vi "test_Expected Response Trigger - S1.vi"(8 "error in (no error)":errorcluster, 11 "TestCase in":refnum<class "Expected Response Trigger test.lvclass">) -> (0 "error out":errorcluster, 3 "TestCase out":refnum<class "Expected Response Trigger test.lvclass">)   [LabVIEW 2017, in "Expected Response Trigger test.lvclass"]
uses:
  Expected Response Trigger test.lvclass
  Libraries/SSH/Expected Response String Config.ctl
  Libraries/SSH/Search Start Point.ctl
  <vilib>/addons/_JKI Toolkits/VI Tester/TestCase.llb/TestCase.lvclass
  Libraries/SSH/SSH.lvlib
  C:/Program Files (x86)/National Instruments/LabVIEW 2017/vi.lib/addons/_JKI Toolkits/VI Tester/TestCase.llb/TestCase.lvclass
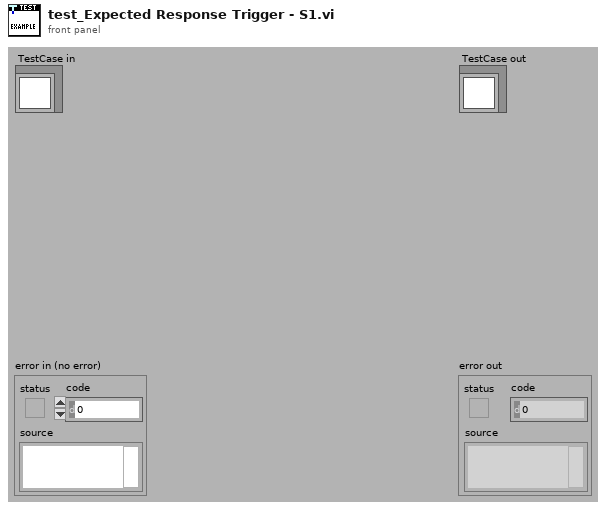
[diagram p1: front panel]
types:
  T1 = typedef "SSH.lvlib/Expected Response String Config.ctl" = cluster{"Expected Response":string, "Search Start Point":T2, "Instance Count":i32}
  T2 = typedef "SSH.lvlib/Search Start Point.ctl" = enum16{"From Start", "From End"}
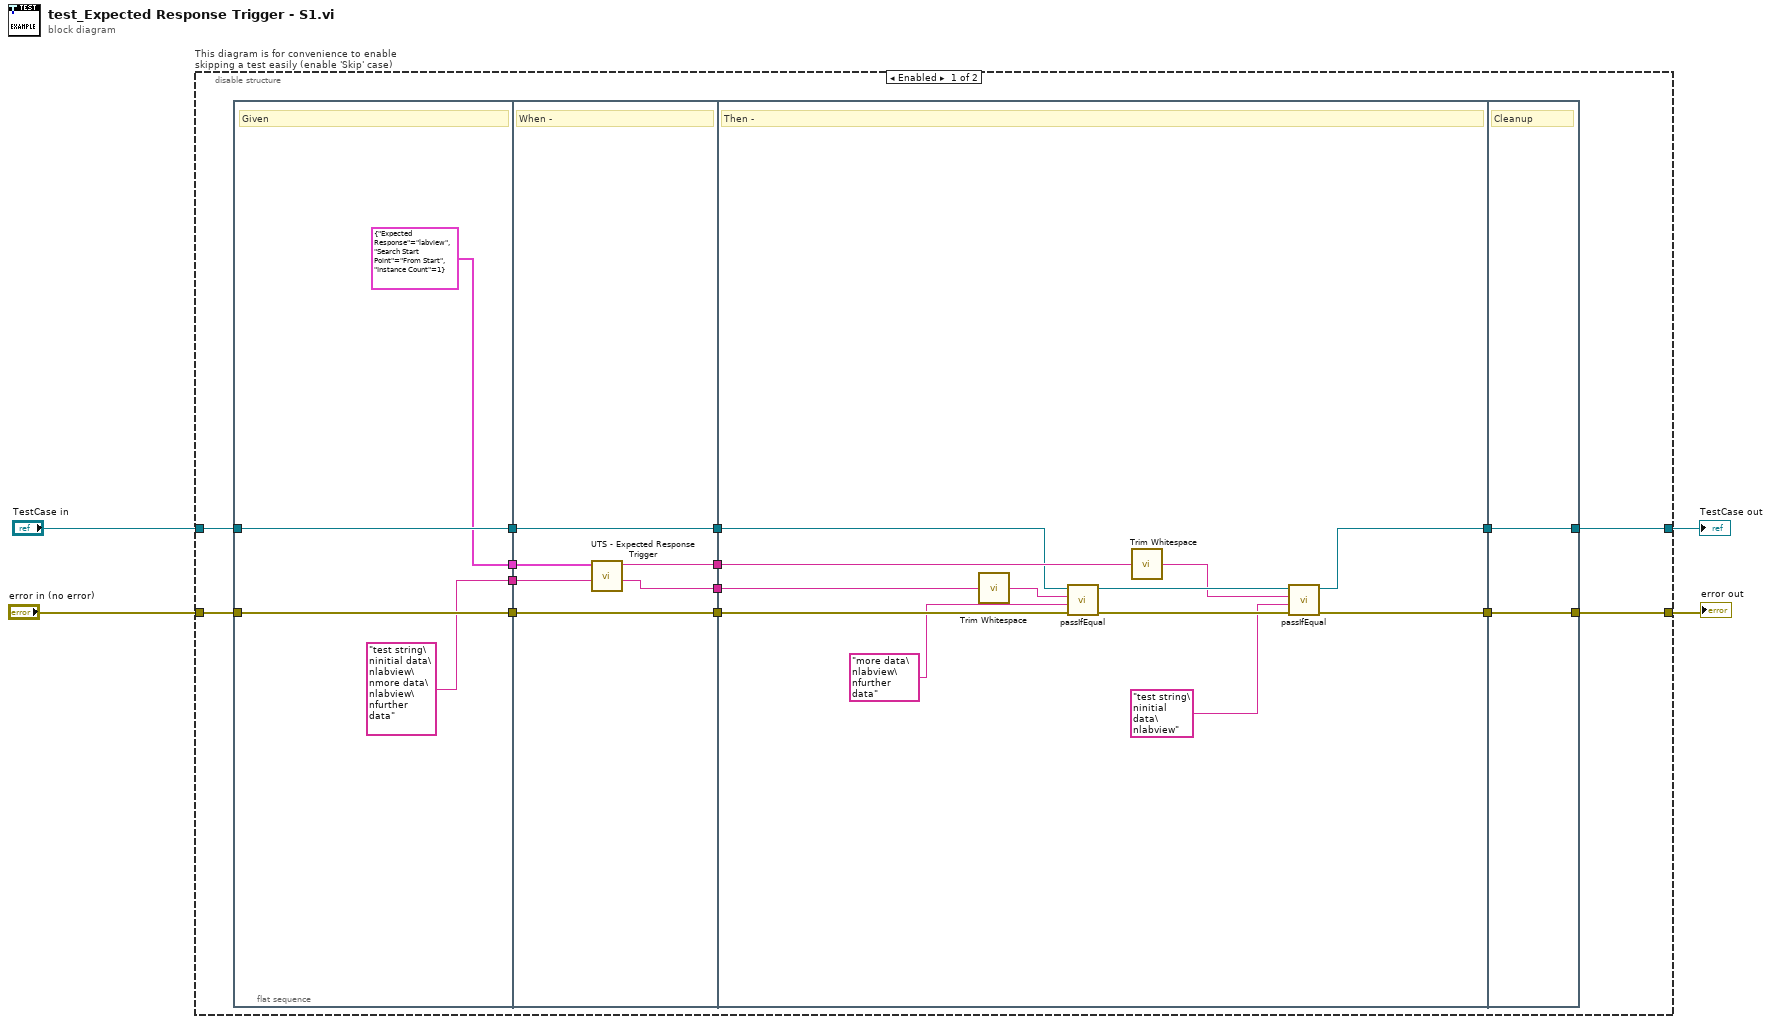
[diagram p0: block diagram]
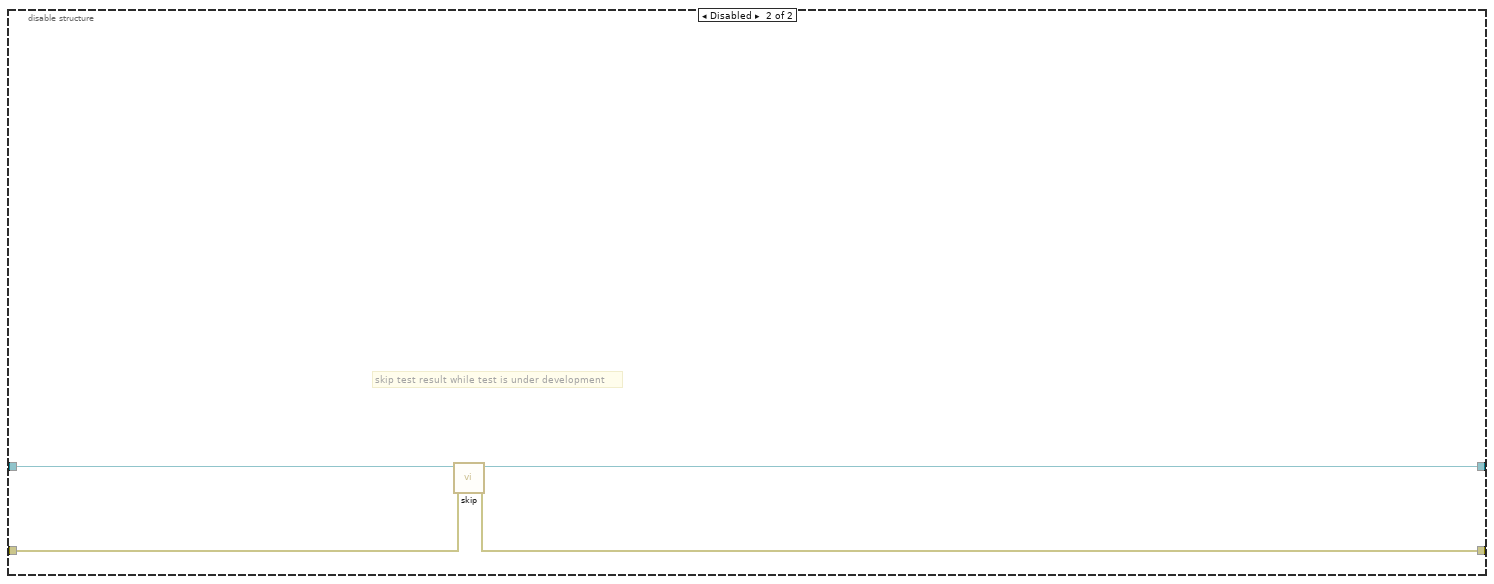
[diagram p2: hidden frame]
diagram:
  n1 = disable-structure "This diagram is for convenience to enable skipping a test easily (enable 'Skip' case)" shown="Enabled" {
    disable-tunnel: "TestCase in" -> [w11 w46]
    disable-tunnel: [w10 w44] -> w1
    disable-tunnel: [w9 w45] -> w3
    disable-tunnel: "error in (no error)" -> [w12 w43]
    frame Enabled {
      n2 = flat-sequence {
        tunnel: w12 -> [w21]
        tunnel: w11 -> [w22]
        tunnel: [w22] -> w18
        tunnel: [w21] -> w17
        tunnel: [T1 {"Expected Response"="labview", "Search Start Point"=enum."From Start", "Instance Count"=1} ("Expected Response String")] -> w8
        tunnel: ["test string\ninitial data\nlabview\nmore data\nlabview\nfurther data" ("String Buffer in")] -> w7
        tunnel: [w28] -> w16
        tunnel: [w27] -> w15
        tunnel: w18 -> [w28]
        tunnel: w17 -> [w27]
        tunnel: w8 -> [w26]
        tunnel: w7 -> [w25]
        tunnel: [w24] -> w6
        tunnel: [w23] -> w5
        tunnel: [w40] -> w14
        tunnel: [w39] -> w13
        tunnel: w16 -> [w37]
        tunnel: w15 -> [w35]
        tunnel: w6 -> [w38]
        tunnel: w5 -> [w36]
        tunnel: [w41] -> w9
        tunnel: [w42] -> w10
        tunnel: w14 -> [w42]
        tunnel: w13 -> [w41]
        frame #0 {
          # "Given"
        }
        frame #1 {
          # "When -"
          n3 = call "UTS - Expected Response Trigger.vi"("String Buffer in"=w25, "Expected Response"=w26) -> ("String Buffer out"=w23:string, "Response"=w24:string)  [unwired: 7 in, 1 out]
        }
        frame #2 {
          # "Then -"
          n4 = call <vilib>:"Trim Whitespace.vi"("string"=w36) -> ("trimmed string"=w32:string)  [unwired: 1 in]
          n5 = call-dynamic "passIfEqual.vi"("error in (no error)"=w35, "y"="more data\nlabview\nfurther data" ("String Buffer in"), "x"=w32, "TestCase in"=w37) -> ("error out"=w34:errorcluster, "TestCase out"=w33:refnum<class "Expected Response Trigger test.lvclass">)  [unwired: 6 in]
          n6 = call <vilib>:"Trim Whitespace.vi"("string"=w38) -> ("trimmed string"=w31:string)  [unwired: 1 in]
          n7 = call-dynamic "passIfEqual.vi"("error in (no error)"=w34, "y"="test string\ninitial data\nlabview" ("String Buffer in"), "x"=w31, "TestCase in"=w33) -> ("error out"=w39:errorcluster, "TestCase out"=w40:refnum<class "Expected Response Trigger test.lvclass">)  [unwired: 6 in]
        }
        frame #3 {
          # "Cleanup"
        }
      }
    }
    frame Disabled {
      # "skip test result while test is under development"
      n8 = call <vilib>:"skip.vi"("error in (no error)"=w43, "TestCase in"=w46) -> ("error out"=w45:errorcluster, "TestCase out"=w44:refnum<class "Expected Response Trigger test.lvclass">)  [unwired: 8 in]
    }
  }
  "error out" <- w3
  "TestCase out" <- w1
